vi "test_Task Actor1.vi"(8 "Error in":errorcluster) -> (0 "error out":errorcluster)   [LabVIEW 2023]
uses:
  <vilib>/ActorFramework/Actor/Actor.lvclass
  Task Actor/Task Actor.lvclass
  Task Base/Task Base.lvclass
  <vilib>/ActorFramework/Stop Msg/Stop Msg.lvclass
  ITask Actor/ITask Actor Messages/Do Msg/Do Msg.lvclass
  Measure and Stimulus Subsystems/Measure and Stimulus Subsystems.lvclass
  C:/Program Files/National Instruments/LabVIEW 2023/vi.lib/ActorFramework/Actor/Actor.lvclass
  D:/git/HAL/HAL GOOP4/Task/Task Actor/Task Actor/Task Actor/Task Actor.lvclass
  D:/git/HAL/HAL GOOP4/Task/Task Actor/ITask Actor/ITask Actor/ITask Actor.lvclass
panel:
  in  "Shutdown Actor":bool
  out "WF Chart":waveform(dbl)(graph)
  out "WF Chart Lossy":waveform(dbl)(graph)
  in  "Stop":bool
  in  "Perform Action":bool
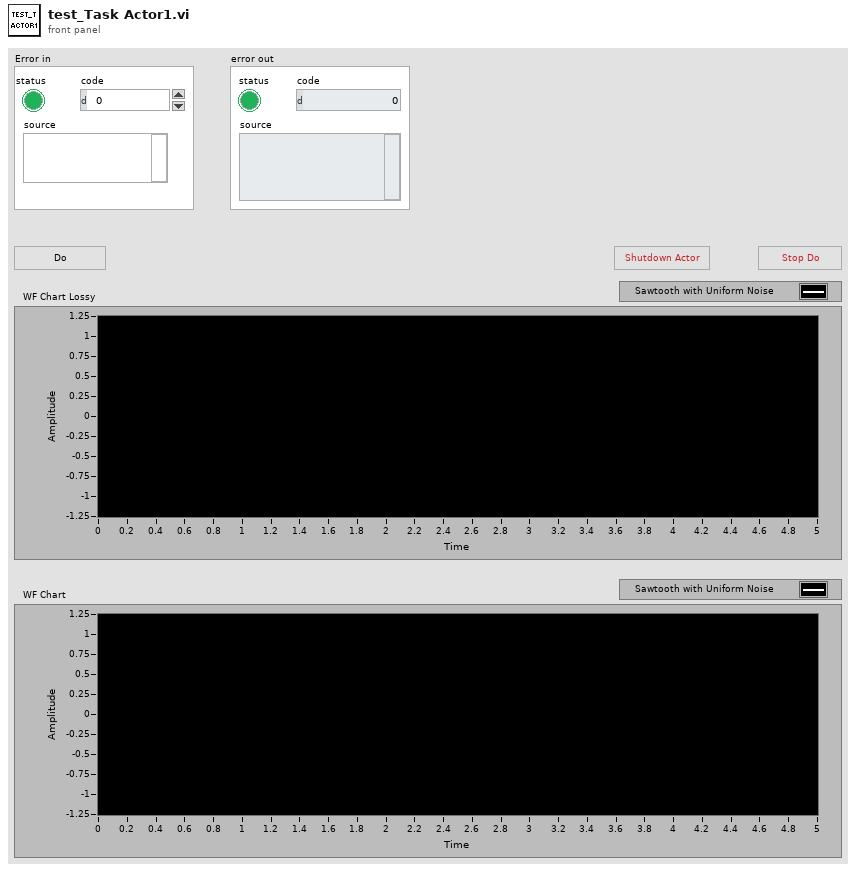
[diagram p1: front panel]
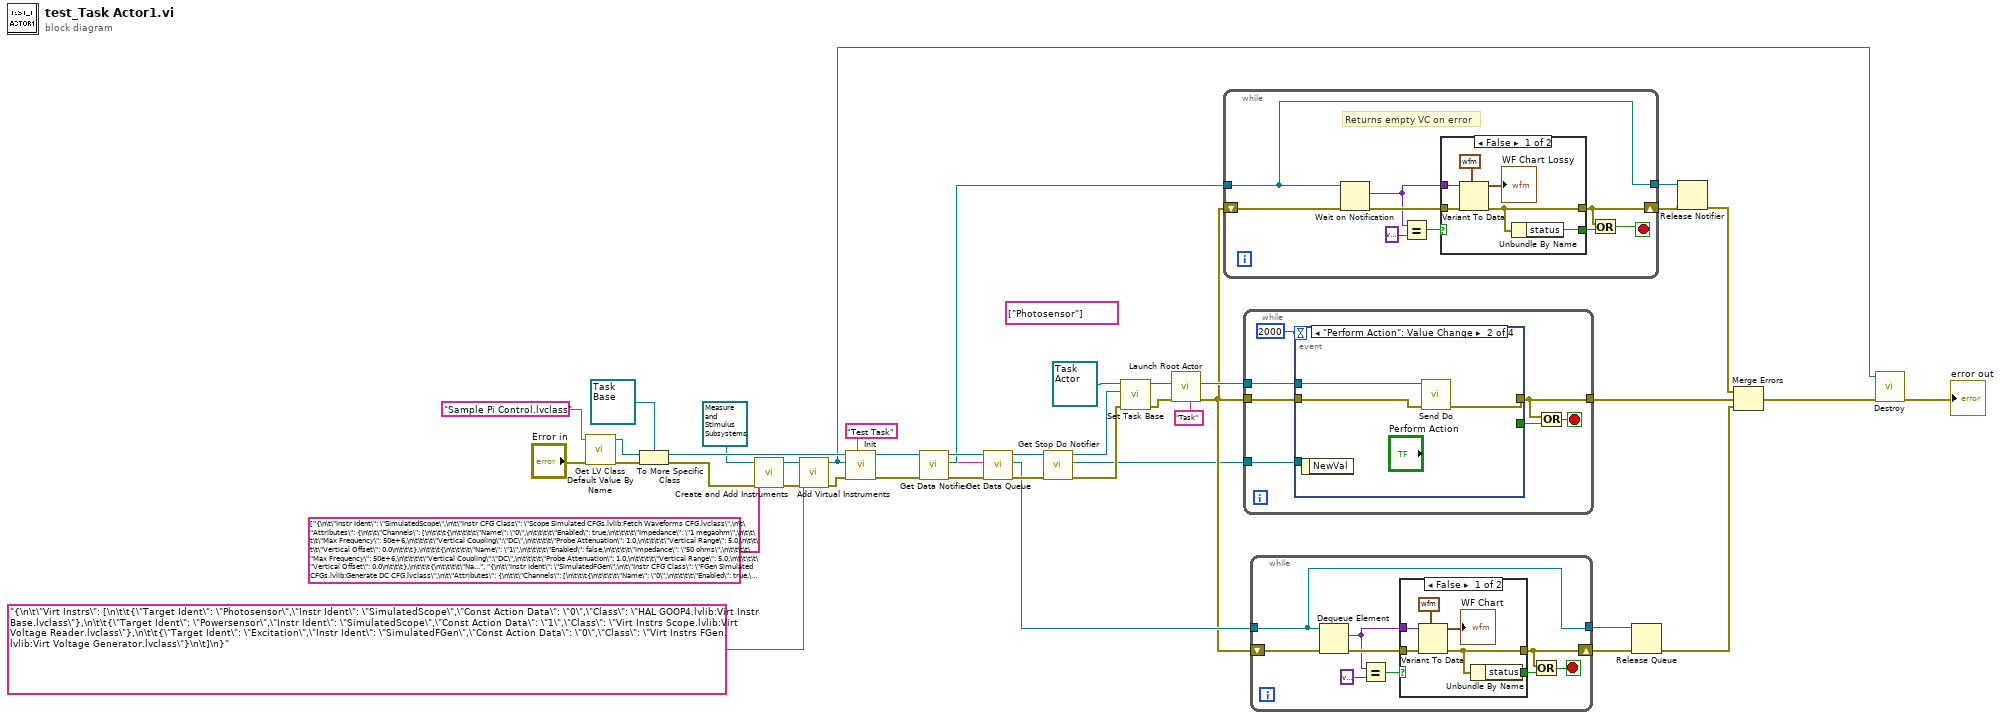
[diagram p0: block diagram]
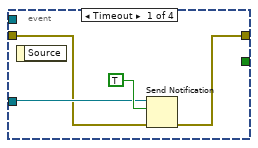
[diagram p4: hidden frame]
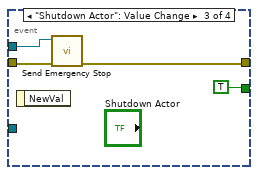
[diagram p5: hidden frame]
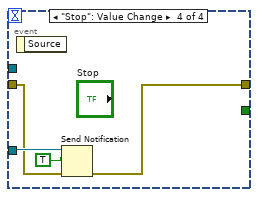
[diagram p6: hidden frame]
diagram:
  (unwired) string[] ["Photosensor"] ("Data Notifier Names")
  n1 = call <vilib>:"Get LV Class Default Value By Name.vi"("error in (no error)"="Error in", "class name"="Sample Pi Control.lvclass") -> ("error out"=w37:errorcluster, "object"=w38:refnum<class>)  [unwired: 8 in]
  n2 = To More Specific Class(target class=refnum<class "Task Base.lvclass"> refnum ("HAL GOOP4.lvlib:Task Base.lvclass"), reference=w38, error in=w37) -> (specific class reference=w35:refnum<class "Task Base.lvclass">, error out=w2:errorcluster)
  n3 = call "Create and Add Instruments.vi"("Error In"=w2, "Physical Intr CFGs"=string[] ["{\n\t\"Instr Ident\": \"SimulatedScope\",\n\t\"Instr CFG Class\": \"Scope Simulated CFGs.lvlib:Fetch Waveforms CFG.lvclass\",\n\t\"Attributes\": {\n\t\t\"Channels\": [\n\t\t\t{\n\t\t\t\t\"Name\": \"0\",\n\t\t\t\t\"Enabled\": true,\n\t\t\t\t\"Impedance\": \"1 megaohm\",\n\t\t\t\t\"Max Frequency\": 50e+6,\n\t\t\t\t\"Vertical Coupling\":\"DC\",\n\t\t\t\t\"Probe Attenuation\": 1.0,\n\t\t\t\t\"Vertical Range\": 5.0,\n\t\t\t\t\"Vertical Offset\": 0.0\n\t\t\t},\n\t\t\t{\n\t\t\t\t\"Name\": \"1\",\n\t\t\t\t\"Enabled\": false,\n\t\t\t\t\"Impedance\": \"50 ohms\",\n\t\t\t\t\"Max Frequency\": 50e+6,\n\t\t\t\t\"Vertical Coupling\":\"DC\",\n\t\t\t\t\"Probe Attenuation\": 1.0,\n\t\t\t\t\"Vertical Range\": 5.0,\n\t\t\t\t\"Vertical Offset\": 0.0\n\t\t\t},\n\t\t\t{\n\t\t\t\t\"Name\": \"2\",\n\t\t\t\t\"Enabled\": false,\n\t\t\t\t\"Impedance\": \"50 ohms\",\n\t\t\t\t\"Max Frequency\": 50e+6,\n\t\t\t\t\"Vertical Coupling\":\"DC\",\n\t\t\t\t\"Probe Attenuation\": 1.0,\n\t\t\t\t\"Vertical Range\": 5.0,\n\t\t\t\t\"Vertical Offset\": 0.0\n\t\t\t},\n\t\t\t{\n\t\t\t\t\"Name\": \"3\",\n\t\t\t\t\"Enabled\": true,\n\t\t\t\t\"Impedance\": \"50 ohms\",\n\t\t\t\t\"Max Frequency\": 50e+6,\n\t\t\t\t\"Vertical Coupling\":\"DC\",\n\t\t\t\t\"Probe Attenuation\": 1.0,\n\t\t\t\t\"Vertical Range\": 1.4,\n\t\t\t\t\"Vertical Offset\": 0.0\n\t\t\t},\n\t\t\t{\n\t\t\t\t\"Name\": \"4\",\n\t\t\t\t\"Enabled\": false,\n\t\t\t\t\"Impedance\": \"50 ohms\",\n\t\t\t\t\"Max Frequency\": 50e+6,\n\t\t\t\t\"Vertical Coupling\":\"DC\",\n\t\t\t\t\"Probe Attenuation\": 1.0,\n\t\t\t\t\"Vertical Range\": 5.0,\n\t\t\t\t\"Vertical Offset\": 0.0\n\t\t\t},\n\t\t\t{\n\t\t\t\t\"Name\": \"5\",\n\t\t\t\t\"Enabled\": false,\n\t\t\t\t\"Impedance\": \"50 ohms\",\n\t\t\t\t\"Max Frequency\": 50e+6,\n\t\t\t\t\"Vertical Coupling\":\"DC\",\n\t\t\t\t\"Probe Attenuation\": 1.0,\n\t\t\t\t\"Vertical Range\": 5.0,\n\t\t\t\t\"Vertical Offset\": 0.0\n\t\t\t},\n\t\t\t{\n\t\t\t\t\"Name\": \"6\",\n\t\t\t\t\"Enabled\": false,\n\t\t\t\t\"Impedance\": \"50 ohms\",\n\t\t\t\t\"Max Frequency\": 50e+6,\n\t\t\t\t\"Vertical Coupling\":\"DC\",\n\t\t\t\t\"Probe Attenuation\": 1.0,\n\t\t\t\t\"Vertical Range\": 5.0,\n\t\t\t\t\"Vertical Offset\": 0.0\n\t\t\t},\n\t\t\t{\n\t\t\t\t\"Name\": \"7\",\n\t\t\t\t\"Enabled\": false,\n\t\t\t\t\"Impedance\": \"50 ohms\",\n\t\t\t\t\"Max Frequency\": 50e+6,\n\t\t\t\t\"Vertical Coupling\":\"DC\",\n\t\t\t\t\"Probe Attenuation\": 1.0,\n\t\t\t\t\"Vertical Range\": 5.0,\n\t\t\t\t\"Vertical Offset\": 0.0\n\t\t\t}\n\t\t],\n\t\t\"Horizontal\": {\n\t\t\t\"Enforce Realtime\": true,\n\t\t\t\"Number of Records\": 1,\n\t\t\t\"Min Sample Rate\": 1e+5,\n\t\t\t\"Reference Position\":50, //percent\n\t\t\t\"Min Record Length\":1e+3\n\t\t},\n\t\t\"Acquire\": {\n\t\t\t\"Type\": \"Normal\",\n\t\t\t\"NumSamples\": 1e+3,\n\t\t\t\"Fetch Relative To\": \"Read Pointer\"\n\t\t},\n\t\t\"Export Signal\": {\n\t\t\t\"Signal Identifier\": \"None\",\n\t\t\t\"Signal\": \"None\",\n\t\t\t\"Output Terminal\": \"None\"\n\t\t},\n\t\t\"Trigger\": {\n\t\t\t\"Type\": \"Immediate\",\n\t\t\t\"Slope\": \"Positive\",\n\t\t\t\"Source\": \"RTSI 0\",\n\t\t\t\"Holdoff\": 0.0,\n\t\t\t\"Delay\": 0.0\n\t\t}\n\t}\n}", "{\n\t\"Instr Ident\": \"SimulatedFGen\",\n\t\"Instr CFG Class\": \"FGen Simulated CFGs.lvlib:Generate DC CFG.lvclass\",\n\t\"Attributes\": {\n\t\t\"Channels\": [\n\t\t\t{\n\t\t\t\t\"Name\": \"0\",\n\t\t\t\t\"Enabled\": true,\n\t\t\t\t\"Waveform\": \"DC\",\n\t\t\t\t\"Frequency\": 0, //DC\n\t\t\t\t\"Amplitude\": 0.0,\n\t\t\t\t\"Start Phase\": 0.0,\n\t\t\t\t\"DC Offset\": 0.0,\n\t\t\t\t\"Trigger Mode\": \"Single\"\n\t\t\t}\n\t\t],\n\t\t\"Export Signal\": {\n\t\t\t\"Enabled\": true,\n\t\t\t\"Output Terminal\": \"PFI 0\",\n\t\t\t\"Signal Identifier\": \"None\",\n\t\t\t\"Signal\": \"Start Trigger\"\n\t\t}\n\t}\n}"], "Host Measure and Stimulus Subsystems in"=refnum<class "Measure and Stimulus Subsystems.lvclass"> refnum) -> ("Error Out"=w34:errorcluster, "Host Measure and Stimulus Subsystems out"=w30:refnum<class "Measure and Stimulus Subsystems.lvclass">)  [unwired: 7 in]
  n4 = call "Add Virtual Instruments.vi"("error in"=w34, "<JSON CFG>"="{\n\t\"Virt Instrs\": [\n\t\t{\"Target Ident\": \"Photosensor\",\"Instr Ident\": \"SimulatedScope\",\"Const Action Data\": \"0\",\"Class\": \"HAL GOOP4.lvlib:Virt Instr Base.lvclass\"},\n\t\t{\"Target Ident\": \"Powersensor\",\"Instr Ident\": \"SimulatedScope\",\"Const Action Data\": \"1\",\"Class\": \"Virt Instrs Scope.lvlib:Virt Voltage Reader.lvclass\"},\n\t\t{\"Target Ident\": \"Excitation\",\"Instr Ident\": \"SimulatedFGen\",\"Const Action Data\": \"0\",\"Class\": \"Virt Instrs FGen.lvlib:Virt Voltage Generator.lvclass\"}\n\t]\n}", "Host Measure and Stimulus Subsystems in"=w30) -> ("error out"=w33:errorcluster, "Host Measure and Stimulus Subsystems out"=w7:refnum<class "Measure and Stimulus Subsystems.lvclass">)  [unwired: 7 in]
  n5 = call-dynamic "Init.vi"("Name"="Test Task", "error in (no error)"=w33, "MSS"=w7, "Task Base in"=w35) -> ("error out"=w29:errorcluster, "Task Base out"=w17:refnum<class "Task Base.lvclass">)  [unwired: 6 in]
  n6 = call "Get Data Notifier.vi"("error in (no error)"=w29, "Target Name"=w10, "Task Base in"=w17) -> ("error out"=w18:errorcluster, "Data Notifier"=w12:refnum<notifier>, "Task Base out"=w15:refnum<class "Task Base.lvclass">)  [unwired: 6 in]
  n7 = call "Get Data Queue.vi"("error in (no error)"=w18, "Task Base in"=w15) -> ("error out"=w16:errorcluster, "Data Queue"=w14:refnum<queue>, "Task Base out"=w5:refnum<class "Task Base.lvclass">, "Target Name"=w10:string)  [unwired: 6 in]
  n8 = call "Get Stop Do Notifier.vi"("error in (no error)"=w16, "Task Base in"=w5) -> ("error out"=w6:errorcluster, "Stop Do"=w3:refnum<notifier>, "Task Base out"=w4:refnum<class "Task Base.lvclass">)  [unwired: 7 in]
  n9 = call "Set Task Base.vi"("error in (no error)"=w6, "HAL GOOP4.lvlib:Task Base.lvclass"=w4, "Task Actor in"=refnum<class "Task Actor.lvclass"> refnum ("Task Actor.lvlib:Task Actor.lvclass")) -> ("error out"=w28:errorcluster, "Task Actor out"=w41:refnum<class "Task Actor.lvclass">)  [unwired: 7 in]
  n10 = call <vilib>:"Launch Root Actor.vi"("Debug Alias"="Task", "error in (no error)"=w28, "Actor"=w41) -> ("error out"=w13:errorcluster, "Actor's Enqueuer"=w27:refnum<class "Message Enqueuer.lvclass">)  [unwired: 7 in]
  n11 = while {
    tunnel: w12 -> [w43]
    shift-right: [w47] -> w24
    shift-left: w13 -> [w49]
    tunnel: [w43] -> w9
    stop <- w48 stop-if-true
    # "Returns empty VC on error"
    n12 = Wait on Notification(notifier=w43, error in (no error)=w49) -> (notification=w50:variant, error out=w51:errorcluster)  [unwired: 2 in, 2 out]
    n13 = Equal?(x=w50, y=variant) -> (x = y?=w45:bool)
    n14 = case shown="False" w45 {
      selector: w45 -> [_ w59]
      tunnel: w51 -> [w57 w58]
      tunnel: [w53 w58] -> w47
      tunnel: w50 -> [w54 _]
      tunnel: [w52 w59] -> w44
      frame False {
        n15 = Variant To Data(error in=w57, type=waveform(dbl) {"t0"=timestamp(0 s since 1904-01-01), "dt"=1.0, "Y"=[]} ("Waveform"), Variant=w54) -> (data=→"WF Chart Lossy":waveform(dbl), error out=w53:errorcluster)
        n16 = Unbundle By Name(w53) -> ("status"=w52:bool)
      }
      frame True {
      }
    }
    n17 = Or(x=w47, y=w44) -> (x .or. y?=w48:bool)
  }
  n18 = while {
    tunnel: w27 -> [w66]
    tunnel: w13 -> [w65]
    tunnel: [w64] -> w25
    tunnel: w3 -> [w61]
    stop <- w63 stop-if-true
    n19 = event shown="[1] \"Perform Action\": Value Change" {
      selector: _ -> [_ _ _ _]
      dyn-events: _ -> [_ _ _ _]
      timeout: 2000 -> [_ _ _ _]
      tunnel: w66 -> [_ w73 w76 _]
      tunnel: w65 -> [w68 w72 w77 w80]
      tunnel: [w67 w71 w75 w78] -> w64
      tunnel: [_ _ TRUE _] -> w62
      tunnel: w61 -> [w69 _ _ w81]
      event Timeout {
        n20 = event-data() -> ()  [unwired: 1 in, 1 out]
        n21 = Send Notification(notification=TRUE, notifier=w69, error in (no error)=w68) -> (error out=w67:errorcluster)  [unwired: 1 out]
      }
      event "Perform Action": Value Change {
        n22 = event-data() -> ()  [unwired: 1 in, 1 out]
        n23 = call "Send Do.vi"("error in (no error)"=w72, "Message Enqueuer"=w73) -> ("error out"=w71:errorcluster)  [unwired: 8 in, 1 out]
      }
      event "Shutdown Actor": Value Change {
        n24 = event-data() -> ()  [unwired: 1 in, 1 out]
        n25 = call <vilib>:"Send Emergency Stop.vi"("error in (no error)"=w77, "Message Enqueuer"=w76) -> ("error out"=w75:errorcluster)  [unwired: 9 in]
      }
      event "Stop": Value Change {
        n26 = event-data() -> ()  [unwired: 1 in, 1 out]
        n27 = Send Notification(notification=TRUE, notifier=w81, error in (no error)=w80) -> (error out=w78:errorcluster)  [unwired: 1 out]
      }
    }
    n28 = Or(x=w64, y=w62) -> (x .or. y?=w63:bool)
  }
  n29 = while {
    tunnel: w14 -> [w85]
    tunnel: [w85] -> w20
    shift-right: [w82] -> w21
    shift-left: w13 -> [w84]
    stop <- w83 stop-if-true
    n30 = Dequeue Element(queue=w85, error in (no error)=w84) -> (element=w89:variant, error out=w90:errorcluster)  [unwired: 1 in, 2 out]
    n31 = Equal?(x=w89, y=variant) -> (x = y?=w87:bool)
    n32 = case shown="False" w87 {
      selector: w87 -> [_ w98]
      tunnel: w90 -> [w96 w97]
      tunnel: [w92 w97] -> w82
      tunnel: w89 -> [w93 _]
      tunnel: [w91 w98] -> w86
      frame False {
        n33 = Variant To Data(error in=w96, type=waveform(dbl) {"t0"=timestamp(0 s since 1904-01-01), "dt"=1.0, "Y"=[]} ("Waveform"), Variant=w93) -> (data=→"WF Chart":waveform(dbl), error out=w92:errorcluster)
        n34 = Unbundle By Name(w92) -> ("status"=w91:bool)
      }
      frame True {
      }
    }
    n35 = Or(x=w82, y=w86) -> (x .or. y?=w83:bool)
  }
  n36 = Release Queue(queue=w20, error in (no error)=w21) -> (error out=w19:errorcluster)  [unwired: 1 in, 2 out]
  n37 = Release Notifier(notifier=w9, error in (no error)=w24) -> (error out=w23:errorcluster)  [unwired: 1 in, 2 out]
  n38 = Merge Errors(w23, w25, w19) -> (w22:errorcluster)
  n39 = call "Destroy.vi"("Error In"=w22, "reference in"=w7) -> ("Error Out"=→"error out":errorcluster)  [unwired: 8 in, 1 out]
